vi "CC lib Range Plus or Minus.vi"(7 "+/- Range":dbl, 9 "Value":dbl, 10 "Target":dbl) -> (1 "In Range?":bool, 2 "coerced(x)":dbl)   [LabVIEW 2021]
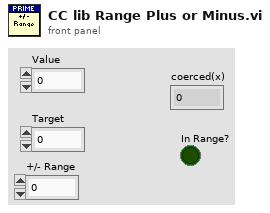
[diagram p1: front panel]
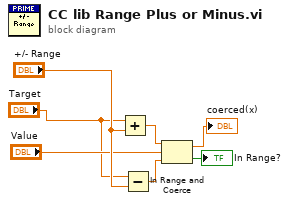
[diagram p0: block diagram]
diagram:
  n1 = Add(x="Target", y="+/- Range") -> (x+y=w7:dbl)
  n2 = Subtract(x="Target", y="+/- Range") -> (x-y=w6:dbl)
  n3 = In Range and Coerce(upper limit=w7, x="Value", lower limit=w6) -> (coerced(x)=→"coerced(x)":dbl, In Range?=→"In Range?":bool)
